vi "To Variant.vi"(0 "TTLDevice in":refnum<class "TTLControlledDevice.lvclass">, 11 "error in (no error)":errorcluster) -> (4 "TTLDevice out":refnum<class "TTLControlledDevice.lvclass">, 8 "Array":variant[](array[variant]), 15 "error out":errorcluster)   [LabVIEW 2020, in "TTLControlledDevice.lvclass"]
uses:
  TTLControlledDevice.lvclass
  D:/Experiment VIs/Koop/KObject Class/KObject.lvclass
  TTLControlledDevice.lvclass/TTLControlledDevice.ctl
  epl-vi-lib/Koop/KObject Class/KObject.lvclass
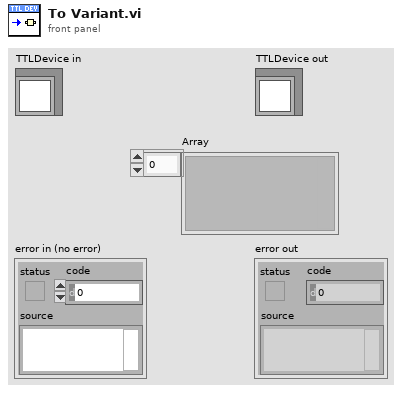
[diagram p1: front panel]
types:
  T1 = typedef "TTLControlledDevice.lvclass/Serialized.ctl" = cluster{"Name":string, "Line":string}
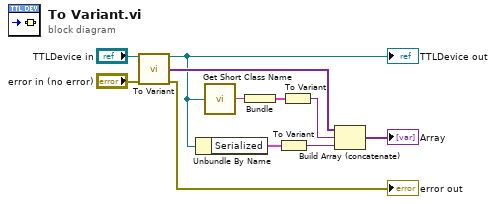
[diagram p0: block diagram]
diagram:
  n1 = call-parent "To Variant.vi"("KObject in"="TTLDevice in", "error in (no error)"="error in (no error)") -> ("KObject out"=w4:refnum<class "TTLControlledDevice.lvclass">, "Array"=w7:variant[], "error out"=→"error out":errorcluster)  [unwired: 11 in]
  "TTLDevice out" <- w4
  n2 = Unbundle By Name(w4) -> ("Serialized"=w8:T1)
  n3 = call "Get Short Class Name.vi"("KObject in"=w4) -> ("Class"=w3:string)  [unwired: 4 in]
  n4 = Bundle("Class"=w3) -> (w2:cluster{"Class":string})  [unwired: 1 in]
  n5 = To Variant(anything=w8) -> (Variant=w5:variant)
  n6 = To Variant(anything=w2) -> (Variant=w1:variant)
  n7 = Build Array (concatenate)(w7, w1, w5) -> (→"Array":variant[])
